vi "1.vi"() -> ()   [LabVIEW 2015]
panel:
  out "Gauge":dbl(knob) scale=0.0..10.0
  in  "Disabled 5":T1(ring)
  in  "Knob":dbl(knob) scale=0.0..10.0
  in  "Path":path
  out "Waveform Chart":dbl(graph)
  in  "Disabled 4":T1(ring)
  out "Tip Strip":string
  out "Description":string
  out "Label.Text":string
  in  "Disabled 3":T1(ring)
  in  "Numeric Control 3":dbl
  out "Cluster 2":cluster{"Knob":dbl, "String":string} {"Knob" scale=0.0..10.0}
  in  "Password":string
  in  "Cluster":cluster{"Knob":dbl, "String":string} {"Knob" scale=0.0..10.0}
  out "Visible 2":bool
  in  "Disabled 2":T1(ring)
  out "Visible":bool
  in  "Numeric Control 2":dbl
  in  "Disabled":T1(ring)
  in  "Numeric Control":dbl
  out "Tank":dbl(slide) scale=0.0..10.0
  in  "Alarm":dbl(slide) scale=0.0..10.0
  in  "Vertical Pointer Slide":dbl(slide) scale=0.0..10.0
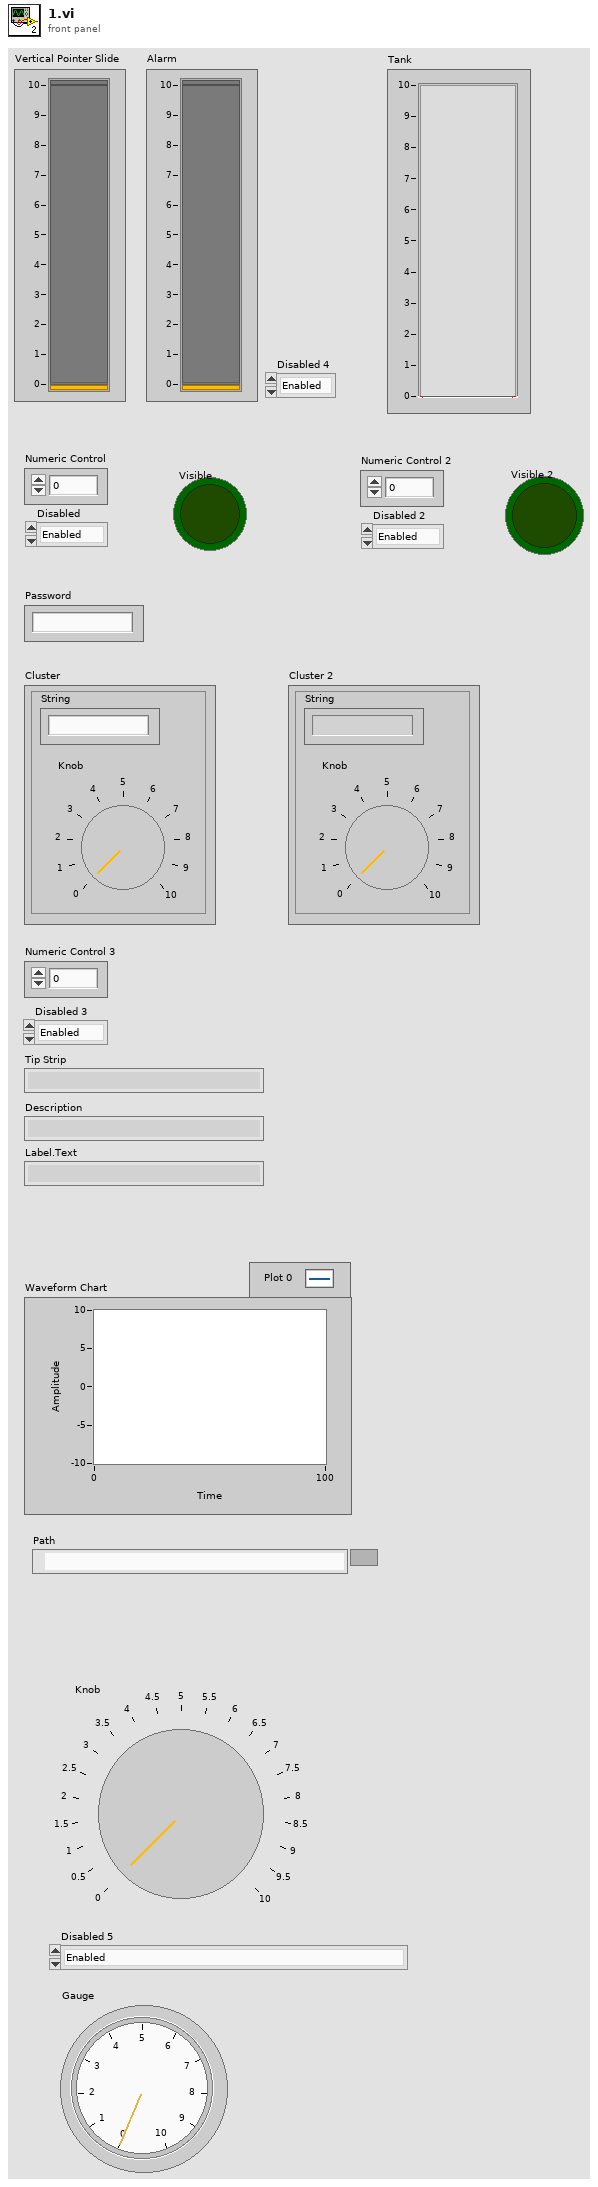
[diagram p1: front panel]
types:
  T1 = enum8{"Enabled", "Disabled", "Disabled and Grayed Out"}
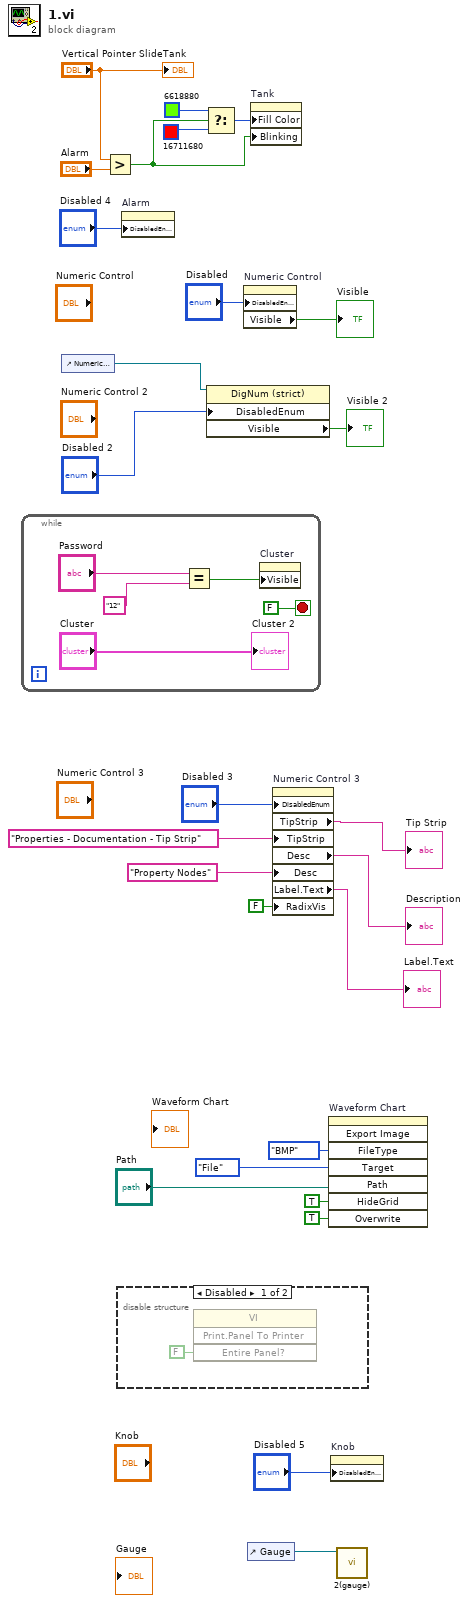
[diagram p0: block diagram]
diagram:
  n1 = while {
    stop <- FALSE stop-if-true
    n2 = Equal?(x="Password", y="12") -> (x = y?=w29:bool)
    n3 = property on="Cluster" class="Clust (strict)"("Visible"=w29) -> ()  [unwired: 2 in, 2 out]
    "Cluster 2" <- "Cluster"
  }
  n4 = control-ref of="Numeric Control 2"() -> (w16:refnum<vi>)
  n5 = Greater?(x="Vertical Pointer Slide", y="Alarm") -> (0:w21:bool)
  n6 = disable-structure shown="Disabled" {
    frame Disabled {
      n7 = invoke class="VI" method="Print.Panel To Printer"("Entire Panel?"=FALSE) -> ()  [unwired: 3 in, 4 out]
    }
    frame Enabled {
    }
  }
  n8 = property on="Alarm" class="Slide (strict)"("DisabledEnum"="Disabled 4") -> ()  [unwired: 2 in, 2 out]
  n9 = Select(t=u32 6618880, s=w21, f=u32 16711680) -> (s? t:f=w23:u32)
  n10 = property on="Property Node" class="DigNum (strict)"(reference=w16, "DisabledEnum"="Disabled 2") -> ("Visible"=→"Visible 2":bool)  [unwired: 1 in, 2 out]
  n11 = property on="Numeric Control" class="DigNum (strict)"("DisabledEnum"="Disabled") -> ("Visible"=→"Visible":bool)  [unwired: 2 in, 2 out]
  n12 = control-ref of="Gauge"() -> (w1:refnum<vi>)
  n13 = property on="Tank" class="Slide (strict)"("Fill Color"=w23, "Blinking"=w21) -> ()  [unwired: 2 in, 2 out]
  n14 = property on="Numeric Control 3" class="DigNum (strict)"("DisabledEnum"="Disabled 3", "TipStrip"="Properties - Documentation - Tip Strip", "Desc"="Property Nodes", "RadixVis"=FALSE ("Radix Visible?")) -> ("TipStrip"=→"Tip Strip":string, "Desc"=→"Description":string, "Label.Text"=→"Label.Text":string)  [unwired: 2 in, 2 out]
  n15 = invoke on="Waveform Chart" class="WFChart (strict)" method="Export Image"("FileType"=enum32{"BMP", "EPS", "EMF", "PICT"}."BMP" ("File Type"), "Target"=enum32{"File", "Clipboard"}."File", "Path"="Path", "HideGrid"=TRUE ("Hide Grid"), "Overwrite"=TRUE ("Always Overwrite")) -> ()  [unwired: 3 in, 8 out]
  n16 = property on="Knob" class="Knob (strict)"("DisabledEnum"="Disabled 5") -> ()  [unwired: 2 in, 2 out]
  n17 = call "2(gauge).vi"("Knob in"=w1) -> ()  [unwired: 11 in]
  "Tank" <- "Vertical Pointer Slide"
